vi "ResetRelEncPos.vi"(0 "error in":errorcluster, 11 "Reset?":bool) -> ()   [LabVIEW 2018]
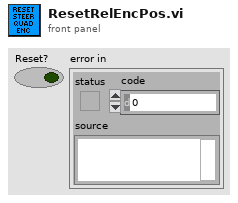
[diagram p1: front panel]
types:
  T1 = typedef "WPI_MotorControlDeviceRef.ctl" = cluster{"DeviceStatus":errorcluster, "Type":T2, "PWM":cluster{"PWM Channel":T3, "DeadBand":T4}, "CAN":cluster{"Device Number":u8, "SetOutput VI Ref":variant, "GetOutput VI Ref":variant, "Enable VI Ref":variant, "Disable VI Ref":variant, "Data":variant}, "Invert":bool, "DIO PWM":cluster{"PWM \"Enable\" Channel":T3, "DIOChannel":T5, "PWM Rate":dbl}}
  T2 = typedef "WPI_MotorControlType.ctl" = enum16{"PWM", "CAN", "DIO PWM"}
  T3 = typedef "FPGA_DIOPWMChannel.ctl" = enum8{"PWM 0", "PWM 1", "PWM 2", "PWM 3", "PWM 4", "PWM 5", "PWM 6", "PWM 7", "PWM 8", "PWM 9", "PWM MXP 0", "PWM MXP 1", "PWM MXP 2", "PWM MXP 3", "PWM MXP 4", "PWM MXP 5", "PWM MXP 6", "PWM MXP 7", "PWM MXP 8", "PWM MXP 9", "Invalid"}
  T4 = typedef "WPI_PWMDeadband.ctl" = cluster{"Name":string, "maxPositivePwm":i32, "minPositivePwm":i32, "centerPwm":i32, "maxNegativePwm":i32, "minNegativePwm":i32, "angularRange":u16}
  T5 = typedef "FPGA_DIOChannel.ctl" = enum8{"DIO 0", "DIO 1", "DIO 2", "DIO 3", "DIO 4", "DIO 5", "DIO 6", "DIO 7", "DIO 8", "DIO 9", "DIO MXP 0", "DIO MXP 1", "DIO MXP 2", "DIO MXP 3", "DIO MXP 4", "DIO MXP 5", "DIO MXP 6", "DIO MXP 7", "DIO MXP 8", "DIO MXP 9", "DIO MXP 10", "DIO MXP 11", "DIO MXP 12", "DIO MXP 13", "DIO MXP 14", "DIO MXP 15", "SPI Port CS1", "SPI Port CS2", "SPI Port CS3", "SPI Port MISO", "SPI Port MOSI", "Invalid"}
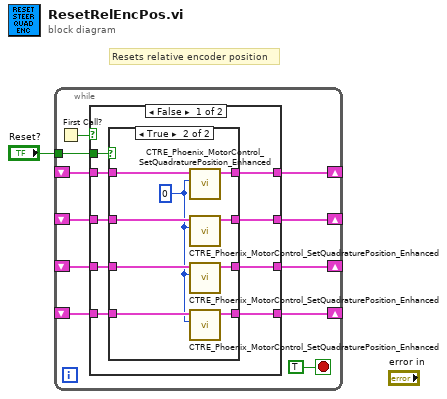
[diagram p0: block diagram]
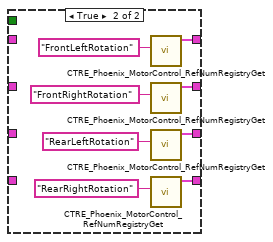
[diagram p3: hidden frame]
diagram:
  # "Resets relative encoder position"
  n1 = while {
    shift-right: [w12] -> _
    shift-left: _ -> [w11]
    tunnel: "Reset?" -> [w9]
    shift-right: [w8] -> _
    shift-left: _ -> [w5]
    shift-right: [w7] -> _
    shift-left: _ -> [w4]
    shift-right: [w6] -> _
    shift-left: _ -> [w3]
    stop <- TRUE stop-if-true
    n2 = First Call?() -> (First Call?: T/F=w10:bool)
    n3 = case shown="False" w10 {
      tunnel: w11 -> [w21 _]
      tunnel: [w20 w38] -> w12
      tunnel: w9 -> [w19 _]
      tunnel: [w17 w37] -> w8
      tunnel: [w16 w36] -> w7
      tunnel: [w13 w35] -> w6
      tunnel: w5 -> [w18 _]
      tunnel: w4 -> [w15 _]
      tunnel: w3 -> [w14 _]
      frame False {
        n4 = case shown="True" w19 {
          tunnel: w21 -> [w25 w34]
          tunnel: [w25 w33] -> w20
          tunnel: w18 -> [w24 w32]
          tunnel: [w24 w31] -> w17
          tunnel: [w23 w30] -> w16
          tunnel: w15 -> [w23 w29]
          tunnel: w14 -> [w22 w28]
          tunnel: [w22 w27] -> w13
          frame False {
          }
          frame True {
            w26 = 0 ("New Position")
            n5 = call <vilib>:"CTRE_Phoenix_MotorControl_SetQuadraturePosition_Enhanced.vi"("New Position"=w26, "PhoenixMotorControlDevRef"=w34) -> ("PhoenixMotorControlDevRef"=w33:T1)  [unwired: 8 in, 1 out]
            n6 = call <vilib>:"CTRE_Phoenix_MotorControl_SetQuadraturePosition_Enhanced.vi"("New Position"=w26, "PhoenixMotorControlDevRef"=w32) -> ("PhoenixMotorControlDevRef"=w31:T1)  [unwired: 8 in, 1 out]
            n7 = call <vilib>:"CTRE_Phoenix_MotorControl_SetQuadraturePosition_Enhanced.vi"("New Position"=w26, "PhoenixMotorControlDevRef"=w29) -> ("PhoenixMotorControlDevRef"=w30:T1)  [unwired: 8 in, 1 out]
            n8 = call <vilib>:"CTRE_Phoenix_MotorControl_SetQuadraturePosition_Enhanced.vi"("New Position"=w26, "PhoenixMotorControlDevRef"=w28) -> ("PhoenixMotorControlDevRef"=w27:T1)  [unwired: 8 in, 1 out]
          }
        }
      }
      frame True {
        n9 = call <vilib>:"CTRE_Phoenix_MotorControl_RefNumRegistryGet.vi"("refnum name"="FrontLeftRotation") -> ("PhoenixMotorControlDevRef"=w38:T1)  [unwired: 9 in, 1 out]
        n10 = call <vilib>:"CTRE_Phoenix_MotorControl_RefNumRegistryGet.vi"("refnum name"="FrontRightRotation") -> ("PhoenixMotorControlDevRef"=w37:T1)  [unwired: 9 in, 1 out]
        n11 = call <vilib>:"CTRE_Phoenix_MotorControl_RefNumRegistryGet.vi"("refnum name"="RearLeftRotation") -> ("PhoenixMotorControlDevRef"=w36:T1)  [unwired: 9 in, 1 out]
        n12 = call <vilib>:"CTRE_Phoenix_MotorControl_RefNumRegistryGet.vi"("refnum name"="RearRightRotation") -> ("PhoenixMotorControlDevRef"=w35:T1)  [unwired: 9 in, 1 out]
      }
    }
  }
